vi "SpecAn Fetch TxP.vi"(0 "Instrument Handle In":refnum<k21>, 1 "Selector String":string, 11 "error in (no error)":errorcluster) -> (4 "Instrument Handle Out":refnum<k21>, 6 "TxP Results":T1 {"Minimum Power (dBm)" format="%.2f"; "Maximum Power (dBm)" format="%.2f"; "Peak to Average Ratio (dB)" format="%.2f"; "Average Mean Power (dBm)" format="%.2f"}, 15 "error out":errorcluster)   [LabVIEW 2016, in "RFmxSpecAn.lvlib"]
doc: "Fetches common results from the TxP measurement."
uses:
  RFmxSpecAn.lvlib
  Typedefs/SpecAn TxP Results.ctl
  <vilib>/RFmx/SpecAn/mx/RFmxSpecAn.llb/RFmxSpecAn TXP Fetch Measurement.vi
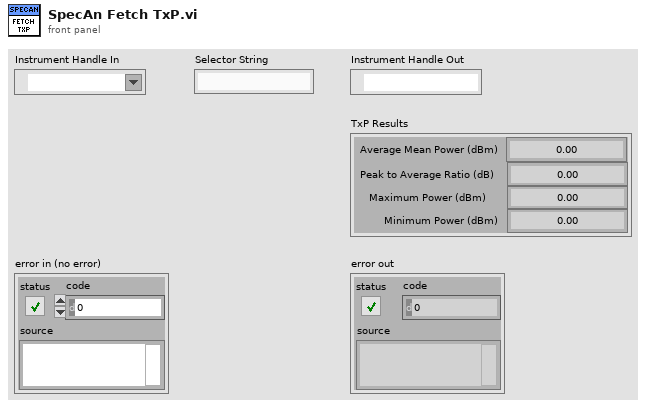
[diagram p1: front panel]
types:
  T1 = typedef "RFmxSpecAn.lvlib/SpecAn TxP Results.ctl" = cluster{"Average Mean Power (dBm)":dbl, "Peak to Average Ratio (dB)":dbl, "Maximum Power (dBm)":dbl, "Minimum Power (dBm)":dbl}
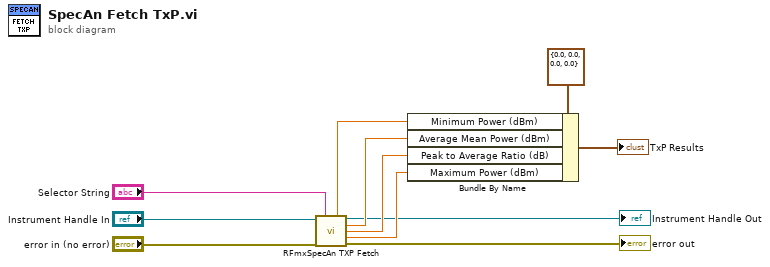
[diagram p0: block diagram]
diagram:
  n1 = call-poly <vilib>:"RFmxSpecAn TXP Fetch.vi"("Instrument Handle In"="Instrument Handle In", "Selector String"="Selector String", "error in (no error)"="error in (no error)") -> ("Minimum Power (dBm)"=w7:dbl, "Instrument Handle Out"=→"Instrument Handle Out":refnum<k21>, "Average Mean Power (dBm)"=w10:dbl, "Peak to Average Ratio (dB)"=w9:dbl, "Maximum Power (dBm)"=w8:dbl, "error out"=→"error out":errorcluster)  [unwired: 7 in]
  n2 = Bundle By Name(cluster=T1 {"Average Mean Power (dBm)"=0.0, "Peak to Average Ratio (dB)"=0.0, "Maximum Power (dBm)"=0.0, "Minimum Power (dBm)"=0.0} ("Cluster"), "Minimum Power (dBm)"=w7, "Average Mean Power (dBm)"=w10, "Peak to Average Ratio (dB)"=w9, "Maximum Power (dBm)"=w8) -> (→"TxP Results":T1)
